vi "process(Client).vi"(8 "error in (no error)":errorcluster, 10 "Sync":refnum<notifier>, 11 "Session in":refnum<class "Session.lvclass">) -> (0 "error out":errorcluster, 3 "Session out":refnum<class "Session.lvclass">)   [LabVIEW 2013]
uses:
  Session.lvclass
panel:
  out "Numeric 3":i32
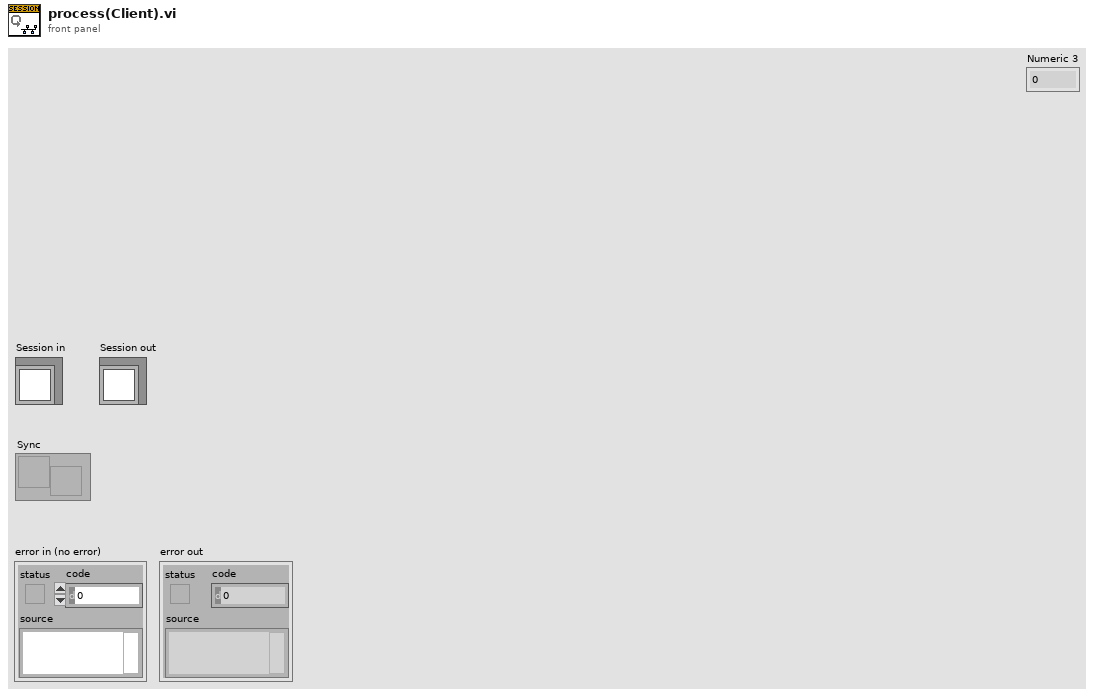
[diagram p1: front panel]
types:
  T1 = typedef "MQTT Base.lvlib/MQTT_Base.lvclass/Response -- cluster.ctl" = cluster{"Packet":refnum<class "ControlPacket.lvclass">, "Protocol Error":errorcluster, "disconnect session":bool, "[ACK]":refnum<notifier>[]}
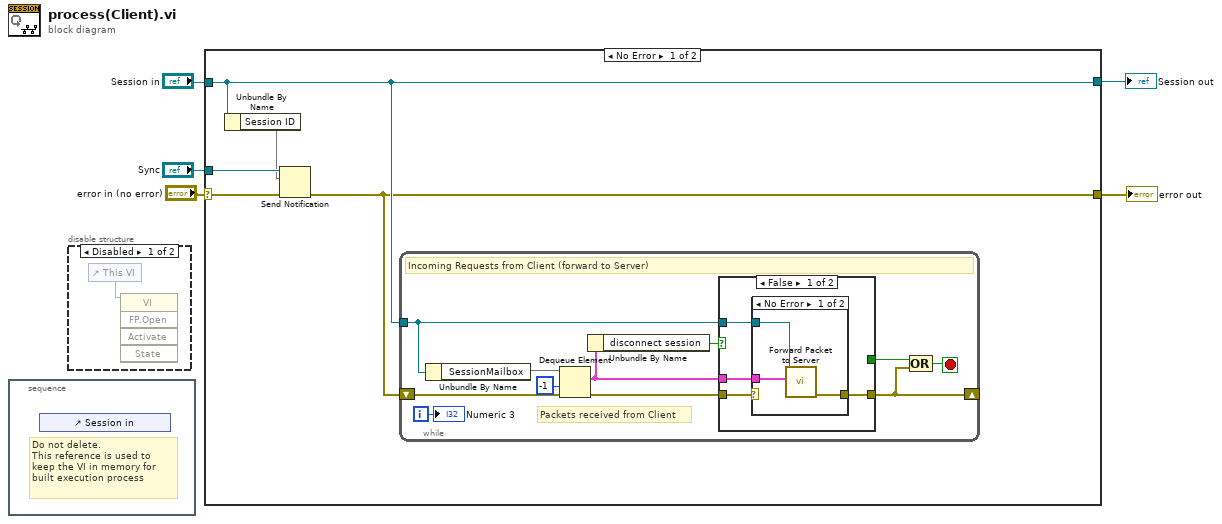
[diagram p0: block diagram]
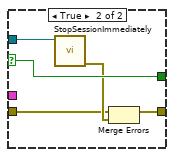
[diagram p4: hidden frame]
diagram:
  n1 = stacked-sequence {
    frame #0 {
      # "Do not delete.\nThis reference is used to keep the VI in memory for built execution process"
      n2 = control-ref of="Session in"() -> ()  [unwired: 1 out]
    }
  }
  n3 = disable-structure shown="Disabled" {
    frame Disabled {
      n4 = control-ref of="This VI"() -> (w6:refnum<vi>)
      n5 = invoke class="VI" method="FP.Open"(reference=w6) -> ()  [unwired: 4 in, 5 out]
    }
    frame Enabled {
    }
  }
  n6 = case shown="No Error" "error in (no error)" {
    selector: "error in (no error)" -> [w10 w37]
    tunnel: [w7 w37] -> w1
    tunnel: [w8 w36] -> w3
    tunnel: "Session in" -> [w8 w36]
    tunnel: "Sync" -> [w11 _]
    frame No Error {
      n7 = Unbundle By Name(w8) -> ("Session ID"=w9)
      n8 = Send Notification(notification=w9, notifier=w11, error in (no error)=w10) -> (error out=w7:errorcluster)  [unwired: 1 out]
      n9 = while {
        tunnel: w8 -> [w18]
        shift-right: [w15] -> _
        shift-left: w7 -> [w19]
        i -> [w13]
        stop <- w14 stop-if-true
        # "Packets received from Client"
        # "Incoming Requests from Client (forward to Server)"
        n10 = Unbundle By Name(w18) -> ("SessionMailbox"=w22)
        n11 = Dequeue Element(queue=w22, timeout in ms (-1)=-1, error in (no error)=w19) -> (element=w17:T1, error out=w20:errorcluster)  [unwired: 2 out]
        n12 = Unbundle By Name(w17) -> ("disconnect session"=w16:bool)
        n13 = case shown="False" w16 {
          selector: w16 -> [_ w35]
          tunnel: w20 -> [w26 w32]
          tunnel: [w25 w31] -> w15
          tunnel: w18 -> [w24 w34]
          tunnel: w17 -> [w23 _]
          tunnel: [_ w35] -> w12
          frame False {
            n14 = case shown="No Error" w26 {
              selector: w26 -> [_ w30]
              tunnel: w23 -> [w28 _]
              tunnel: [w27 w30] -> w25
              tunnel: w24 -> [w29 _]
              frame No Error {
                n15 = call "Forward Packet to Server.vi"("Message"=w28, "Session in"=w29) -> ("error out"=w27:errorcluster)  [unwired: 9 in]
              }
              frame Error {
              }
            }
          }
          frame True {
            n16 = call "StopSessionImmediately.vi"("Session in"=w34) -> ("error out"=w33:errorcluster)  [unwired: 9 in, 1 out]
            n17 = Merge Errors(w32, w33) -> (w31:errorcluster)
          }
        }
        n18 = Compound Arithmetic op=OR(w12, w15) -> (w14:bool)
        "Numeric 3" <- w13
      }
    }
    frame Error {
    }
  }
  "error out" <- w1
  "Session out" <- w3
